vi "SpecialChs.vi"(1 "Ain?":bool, 2 "mV low":i32[](array[numeric])=[0, 0, 0, 0, 0, 0, 0, 0, 0, 0, 0, 0, 0, 0, 0, 0, 0, 0, 0, 0, 0, 0, 0, 0, 0, 0, 0, 0, 0, 0, 0, 0, 0, 0, 0, 0, 0, 0, 0, 0, 0, 0, 0, 0, 0, 0, 0, 0]) -> (0 "mV low New":i32[](array[numeric]))   [LabVIEW 2011]
uses:
  Globals/SysGlbs.vi
  11805/SpecGlbs.vi
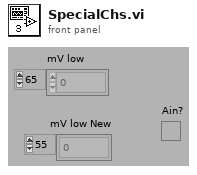
[diagram p1: front panel]
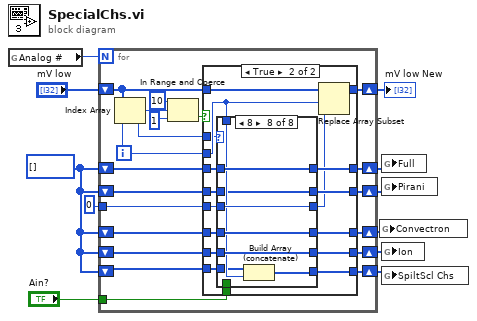
[diagram p0: block diagram]
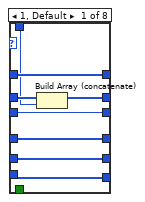
[diagram p3: hidden frame]
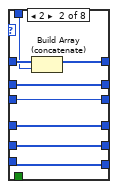
[diagram p4: hidden frame]
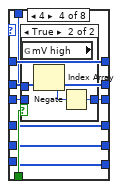
[diagram p6: hidden frame]
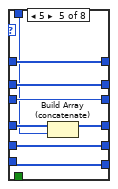
[diagram p8: hidden frame]
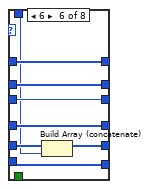
[diagram p9: hidden frame]
diagram:
  w1 = i32[] []
  n1 = global read "SysGlbs.vi" "Analog #"() -> (w11:u32)
  n2 = for {
    N: w11 -> [_]
    shift-right: [w26] -> w9
    shift-left: "mV low" -> [w27]
    shift-right: [w24] -> w7
    shift-left: w1 -> [w25]
    shift-right: [w22] -> w8
    shift-left: w1 -> [w23]
    tunnel: 0 -> [w20]
    tunnel: "Ain?" -> [w19]
    shift-right: [w17] -> w4
    shift-left: w1 -> [w18]
    shift-right: [w15] -> w3
    shift-left: w1 -> [w16]
    shift-right: [w13] -> w2
    shift-left: w1 -> [w12]
    i -> [w30]
    n3 = Index Array(array=w27, index=w30) -> (element=w21:i32)
    n4 = In Range and Coerce(upper limit=10, x=w21, lower limit=1) -> (In Range?=w28:bool)  [unwired: 1 out]
    n5 = case shown="True" w28 {
      tunnel: w27 -> [w36 w53]
      tunnel: [w36 w52] -> w26
      tunnel: w30 -> [_ w48]
      tunnel: w25 -> [w35 w51]
      tunnel: [w35 w50] -> w24
      tunnel: w23 -> [w34 w49]
      tunnel: [w34 w46] -> w22
      tunnel: w21 -> [_ w47]
      tunnel: w20 -> [_ w45]
      tunnel: w19 -> [_ w43]
      tunnel: w18 -> [w33 w42]
      tunnel: [w33 w41] -> w17
      tunnel: w16 -> [w32 w40]
      tunnel: [w32 w39] -> w15
      tunnel: [w31 w38] -> w13
      tunnel: w12 -> [w31 w37]
      frame False {
      }
      frame True {
        n6 = case shown="8" w47 {
          tunnel: w51 -> [w61 w69 w75 w84 w97 w105 w111 w119]
          tunnel: [w61 w68 w75 w84 w97 w105 w111 w119] -> w50
          tunnel: w49 -> [w60 w67 w74 w83 w96 w104 w110 w112]
          tunnel: w48 -> [w59 w66 _ w79 w93 w99 _ w115]
          tunnel: [w58 w67 w74 w83 w96 w104 w110 w112] -> w46
          tunnel: w45 -> [w57 w65 w73 w81 w95 w102 w109 w118]
          tunnel: [w57 w65 w73 w80 w95 w102 w109 w118] -> w44
          tunnel: w43 -> [_ _ _ w82 _ _ _ _]
          tunnel: w42 -> [w56 w64 w72 w78 w94 w103 w108 w117]
          tunnel: [w56 w64 w72 w78 w92 w103 w108 w117] -> w41
          tunnel: w40 -> [w55 w63 w71 w77 w91 w101 w107 w116]
          tunnel: [w55 w63 w71 w77 w91 w100 w107 w116] -> w39
          tunnel: [w54 w62 w70 w76 w90 w98 w106 w113] -> w38
          tunnel: w37 -> [w54 w62 w70 w76 w90 w98 w106 w114]
          frame 1, Default {
            n7 = Build Array (concatenate)(w60, w59) -> (w58:i32[])
          }
          frame 2 {
            n8 = Build Array (concatenate)(w69, w66) -> (w68:i32[])
          }
          frame 3 {
          }
          frame 4 {
            n9 = case shown="True" w82 {
              tunnel: w81 -> [w85 _]
              tunnel: [w85 w86] -> w80
              tunnel: w79 -> [_ w88]
              frame False {
              }
              frame True {
                n10 = global read "SysGlbs.vi" "mV high"() -> (w89:i32[])
                n11 = Index Array(array=w89, index=w88) -> (element=w87:i32)
                n12 = Negate(x=w87) -> (-x=w86:i32)
              }
            }
          }
          frame 5 {
            n13 = Build Array (concatenate)(w94, w93) -> (w92:i32[])
          }
          frame 6 {
            n14 = Build Array (concatenate)(w101, w99) -> (w100:i32[])
          }
          frame 7 {
          }
          frame 8 {
            n15 = Build Array (concatenate)(w114, w115) -> (w113:i32[])
          }
        }
        n16 = Replace Array Subset(array=w53, new element=w44, index=w48) -> (w52:i32[])
      }
    }
  }
  "mV low New" <- w9
  n17 = global write "SysGlbs.vi" "Convectron"(w4) -> ()
  n18 = global write "SysGlbs.vi" "Full"(w7) -> ()
  n19 = global write "SysGlbs.vi" "Pirani"(w8) -> ()
  n20 = global write "SysGlbs.vi" "Ion"(w3) -> ()
  n21 = global write "SpecGlbs.vi" "SpiltScl Chs"(w2) -> ()
